vi "服务器.vi"() -> ()   [LabVIEW 2017]
panel:
  in  "停止":bool
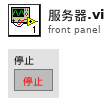
[diagram p1: front panel]
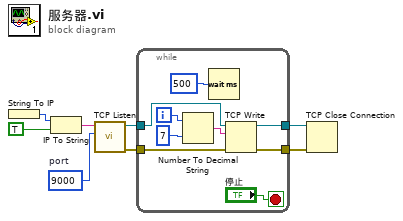
[diagram p0: block diagram]
diagram:
  w8 = u16 9000  # port
  n1 = String To IP() -> (0:w6:u32)  [unwired: 1 in]
  n2 = IP To String(1:TRUE ("句点符号？(F)"), 2:w6) -> (0:w5:string)
  n3 = call <vilib>:"TCP Listen.vi"("port"=w8, "service name"=w5) -> ("error out"=w3:errorcluster, "connection ID"=w4:refnum<k5>)  [unwired: 5 in, 3 out]
  n4 = while {
    tunnel: w4 -> [w17]
    tunnel: w3 -> [w16]
    tunnel: [w15] -> w2
    tunnel: [w14] -> w1
    i -> [w11]
    stop <- "停止" stop-if-true
    n5 = Number To Decimal String(number=w11, width (-)=i16 7 ("宽度(-)")) -> (decimal integer string=w10:string)
    n6 = Wait (ms)(milliseconds to wait=u32 500 ("等待时间（毫秒）")) -> ()  [unwired: 1 out]
    n7 = TCP Write(connection ID=w17, data in=w10, error in (no error)=w16) -> (connection ID out=w15:refnum<k5>, error out=w14:errorcluster)  [unwired: 1 in, 1 out]
  }
  n8 = TCP Close Connection(connection ID=w2, error in (no error)=w1) -> ()  [unwired: 1 in, 2 out]
